vi "UDP Client.vi"() -> ()   [LabVIEW 2009]
doc: "This VI implements a client for the Named Service UDP Server.vi.\nIt connects to a service by specifying the server address and the name of the service. After sending a 'Hello' string to the server, the client receives the string sent by the server, displays the string and closes the connection.\n\n<b>Note:</b> This VI is built to work with the Named Service UDP Server.vi in UDP.llb."
panel:
  out "data out":string
  out "error out":errorcluster
  in  "error in":errorcluster
  # "Instructions:\n1. Open Named Service UDP Server.vi located in the same library.\n2. Follow the instructions on it's front panel.\n\nNote: This VI is built to work with the Named Service UDP Server.vi in UDP.llb."
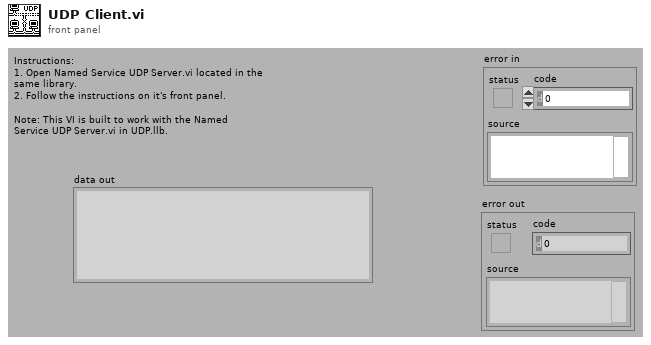
[diagram p1: front panel]
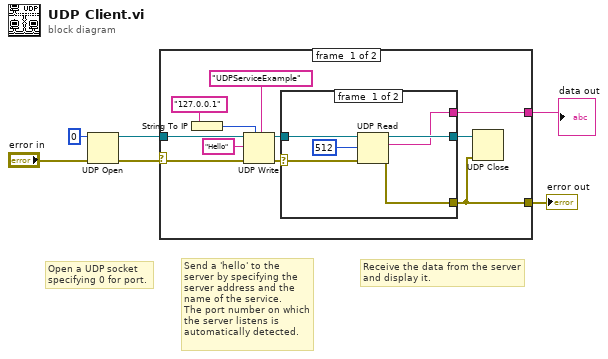
[diagram p0: block diagram]
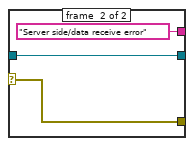
[diagram p2: hidden frame]
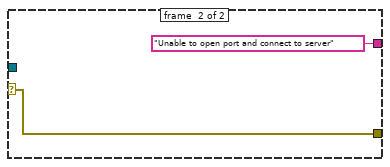
[diagram p3: hidden frame]
diagram:
  # "Receive the data from the server\nand display it."
  # "Send a 'hello' to the\nserver by specifying the\nserver address and the\nname of the service.\nThe port number on which \nthe server listens is\nautomatically detected."
  # "Open a UDP socket\nspecifying 0 for port."
  n1 = UDP Open(8:"error in", 11:0) -> (port=w2:refnum<k16>, 0:w3:errorcluster)  [unwired: 3 in, 1 out]
  n2 = case shown="No Error" w3 {
    selector: w3 -> [w17 w28]
    tunnel: [w9 w28] -> w6
    tunnel: w2 -> [w16 _]
    tunnel: [w7 "Unable to open port and connect to server" ("data out")] -> w1
    frame #0 {
      n3 = String To IP(1:"127.0.0.1") -> (0:w14:u32)
      n4 = UDP Write(address=w14, port or service name="UDPServiceExample", connection ID=w16, data in="Hello", 8:w17) -> (error out=w12:errorcluster, 3:w11:refnum<k16>)  [unwired: 1 in]
      n5 = case shown="No Error" w12 {
        selector: w12 -> [w23 w25]
        tunnel: w11 -> [w22 w26]
        tunnel: [w20 w26] -> w10
        tunnel: [w19 w25] -> w9
        tunnel: [w18 "Server side/data receive error" ("data out")] -> w7
        frame #0 {
          n6 = UDP Read(connection ID=w22, max size (548)=512, 8:w23) -> (data out=w18:string, error out=w19:errorcluster, 3:w20:refnum<k16>)  [unwired: 1 in, 2 out]
        }
        frame #1 {
        }
      }
      n7 = UDP Close(connection ID=w10, 8:w9) -> ()  [unwired: 2 out]
    }
    frame #1 {
    }
  }
  "error out" <- w6
  "data out" <- w1
